vi "Motor_Plus_Impedance_controller.vi"() -> ()   [LabVIEW 2016]
uses:
  <vilib>/Platform/TimedLoop/XDataNode/timing_clust.ctl
  <vilib>/Platform/TimedLoop/XDataNode/nitl_modes.ctl
  <vilib>/Platform/TimedLoop/XDataNode/wakeup.ctl
  <vilib>/Platform/TimedLoop/XDataNode/loadnilvce.vi
  <vilib>/Motion/Express/_s/nimc.ax.power.power.axis.vi
  <vilib>/Motion/Express/_s/nimc.fb.stopMove.stop.axis.modeDecelerate.vi
  <vilib>/Motion/Express/_s/nimc.fb.read.readExecutionData.axis.vi
  <vilib>/Motion/Express/_s/nimc.fb.straightLineMove.startStraightLineMove.axis.modeAbsolute.0.vi
  <vilib>/Motion/Express/_s/nimc.ex.power.power.axis.vi
  <vilib>/platform/TimedLoop/XDataNode/XDataNode.xnode
  <vilib>/Motion/BlockNode/FB.NIMotion.xnode
  <vilib>/Platform/TimedLoop/XDataNode/XDNodeRunTimeDep.lvlib
panel:
  out "Torque":dbl(knob) scale=0.0..10.0
  out "Position":dbl(knob) scale=0.0..10.0
  out "Velocity":dbl(knob) scale=0.0..10.0
  out "Load Cell":dbl(knob) scale=0.0..10.0
  in  "desired motor\nposition":dbl
  in  "Move to Position?":bool
  out "Load cell, V":dbl format="%.3f"
  out "motor torque, Nm":dbl format="%.3f"
  out "motor velocity, rev/s":dbl format="%.3f"
  out "motor position, rev":dbl format="%.3f"
  in  "STOP VI":bool
  in  "Enable Axis \nControl":bool
  in  "Enable Motor \nDrive":bool
  in  "EMERGENCY MOTOR STOP":bool
  # "Raw Data from System"
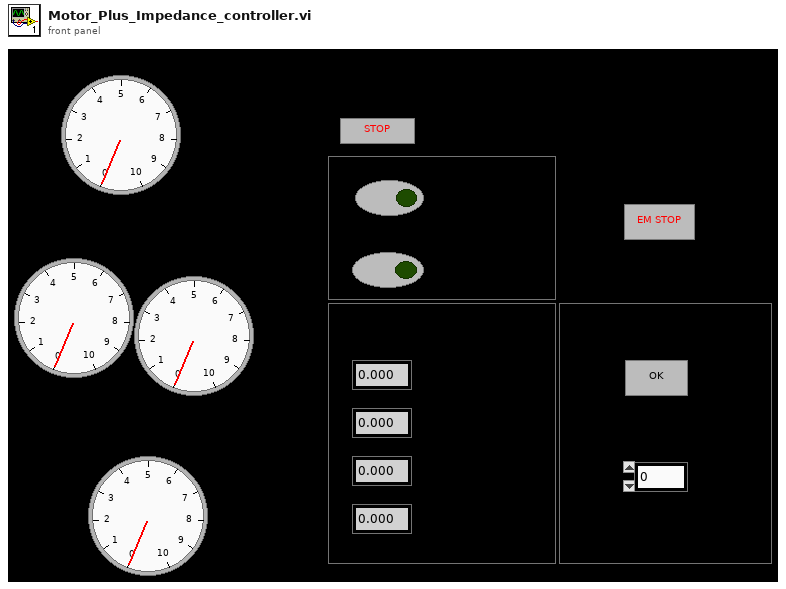
[diagram p1: front panel]
types:
  T1 = typedef "XDNodeRunTimeDep.lvlib/timing_clust.ctl" = cluster{"Expected End [f-1]":u64, "Actual End [f-1]":u64, "Finished Late? [f-1]":bool, "Expected End [i-1]":u64, "Actual End [i-1]":u64, "Finished Late? [i-1]":bool, "Expected Start [i]":u64, "Actual Start [i]":u64, "Expected Start [f]":u64, "Actual Start [f]":u64, "Source Name":string, "Structure Name":string, "Period":i64, "Deadline":i64, "Offset":i64, "Start":i64, "Priority":i32, "Timeout":i32, "Mode":T2, "Wakeup Reason":T3, "Error":errorcluster, "Source Type":string, "Secondary Source Type":string, "Global End Time":u64, "Global Start Time":u64, "Frame Duration":u64, "Iteration Duration":u64, "Assigned CPU":i32, "I/O Scan Engine Mode":u32}
  T2 = typedef "XDNodeRunTimeDep.lvlib/nitl_modes.ctl" = enum32{"No Change", "Process missed periods, maintain original phase", "Discard missed periods, maintain original phase", "Process missed periods, ignore original phase", "Discard missed periods, ignore original phase"}
  T3 = typedef "XDNodeRunTimeDep.lvlib/wakeup.ctl" = enum32{"Normal", "Aborted", "Asynchronous wakeup", "Timing source error", "Timed loop error", "Timeout"}
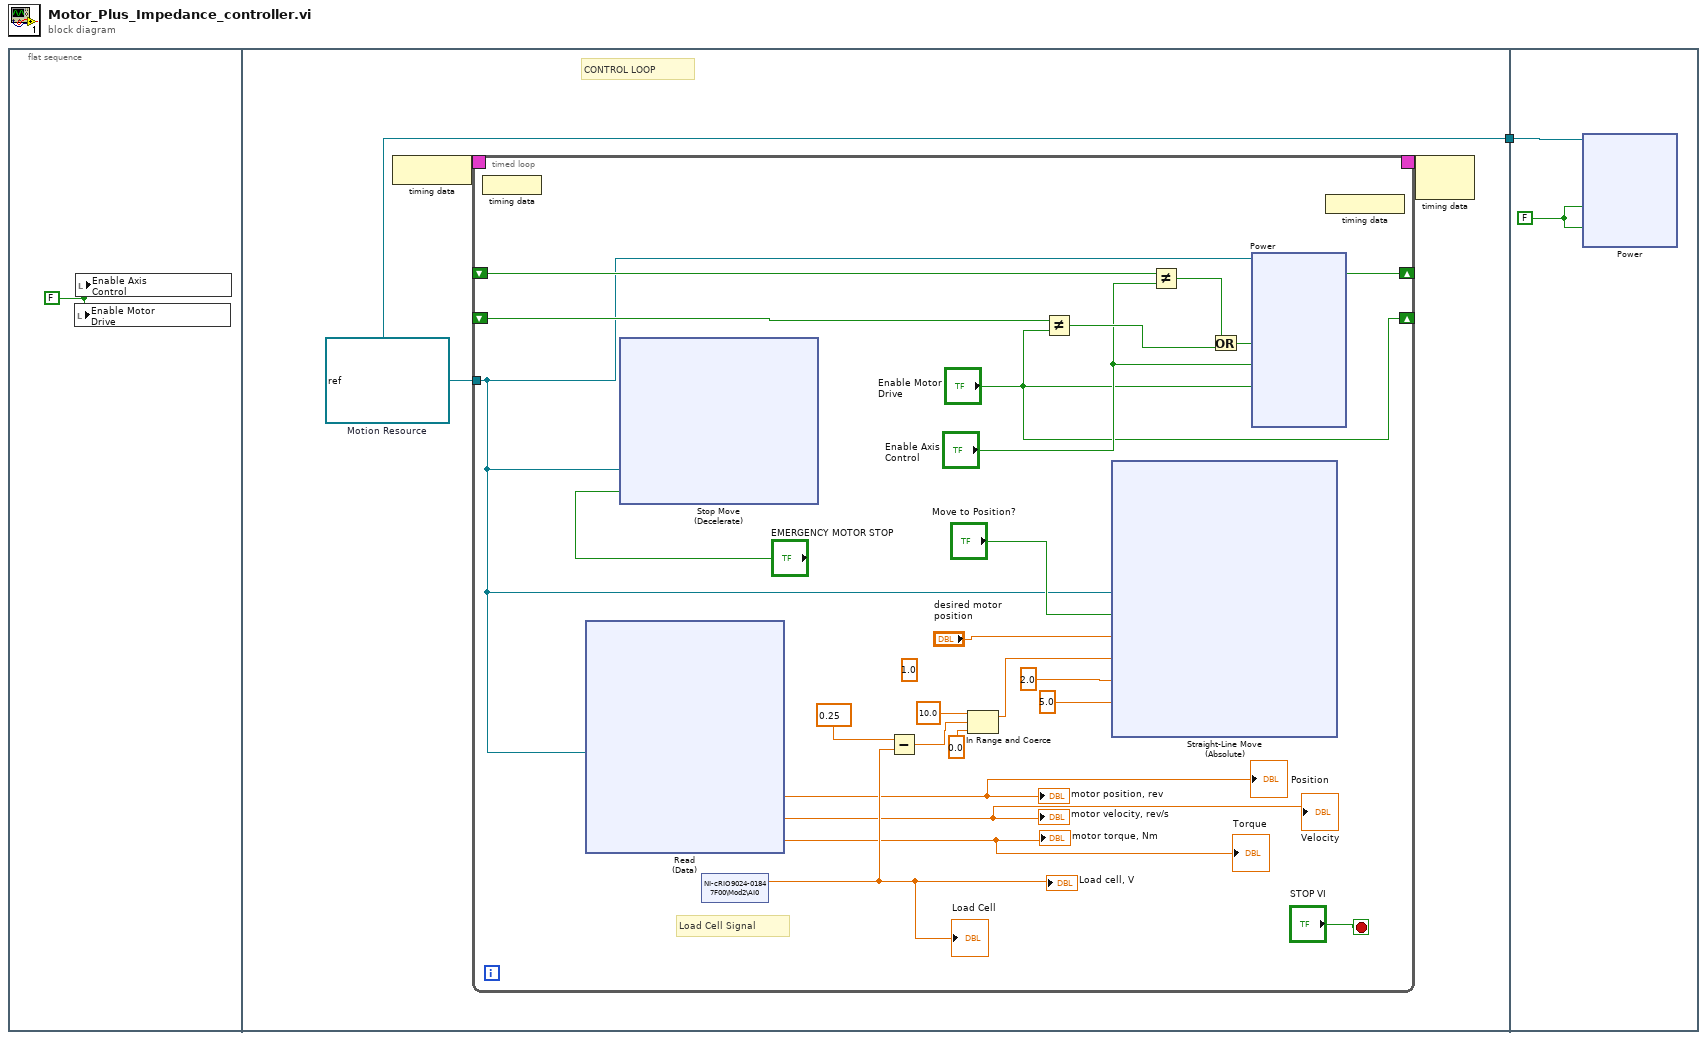
[diagram p0: block diagram]
diagram:
  n1 = flat-sequence {
    tunnel: [w5] -> w1
    tunnel: w1 -> [w96]
    frame #0 {
      w2 = FALSE
      n2 = local write "Enable Motor \nDrive"(w2) -> ()
      n3 = local write "Enable Axis \nControl"(w2) -> ()
    }
    frame #1 {
      w5 = refnum<k21> "nism://NI-cRIO9024-01847F00/Axis 1"  # Motion Resource
      # "CONTROL LOOP"
      n4 = node-c288() -> (w4:T1)
      n5 = timed-loop {
        tunnel: w5 -> [w16]
        timing: w4 -> [_]
        timing-out: [_] -> w3
        shift-right: ["Enable Axis \nControl"] -> _
        shift-left: _ -> [w24]
        shift-right: ["Enable Motor \nDrive"] -> _
        shift-left: _ -> [w23]
        stop <- "STOP VI" stop-if-true
        (unwired) 1.0
        # "Load Cell Signal"
        n6 = node-c288() -> ()  [unwired: 1 in]
        n7 = xnode "Read\n(Data)"("resource"=w16) -> ("position"=→"motor position, rev" →"Position":dbl, "torque"=→"motor torque, Nm" →"Torque":dbl, "velocity"=→"motor velocity, rev/s" →"Velocity":dbl)  [unwired: 1 in, 3 out]
        n8 = xnode "Stop Move\n(Decelerate)"("resource"=w16, "execute"="EMERGENCY MOTOR STOP") -> ()  [unwired: 1 in, 3 out]
        n9 = shared-variable "NI-cRIO9024-01847F00\\Mod2\\AI0"() -> (w9:dbl)  [unwired: 1 in, 1 out]
        "Load cell, V" <- w9
        "Load Cell" <- w9
        n10 = Subtract(x=0.25, y=w9) -> (x-y=w11:dbl)
        n11 = In Range and Coerce(upper limit=10.0, x=w11, lower limit=0.0) -> (coerced(x)=w10:dbl)  [unwired: 1 out]
        n12 = Not Equal?(x=w23, y="Enable Motor \nDrive") -> (x != y?=w21:bool)
        n13 = xnode "Straight-Line Move\n(Absolute)"("resource"=w16, "execute"="Move to Position?", "position"="desired motor\nposition", "velocity"=w10, "acceleration"=2.0, "deceleration"=5.0) -> ()  [unwired: 1 in, 3 out]
        n14 = Not Equal?(x=w24, y="Enable Axis \nControl") -> (x != y?=w22:bool)
        n15 = Or(x=w22, y=w21) -> (x .or. y?=w20:bool)
        n16 = xnode ("Power")("execute"=w20, "enable axis"="Enable Axis \nControl", "enable drive"="Enable Motor \nDrive", "resource"=w16) -> ()  [unwired: 1 in, 6 out]
        n17 = node-c288() -> ()  [unwired: 1 out]
      }
      n18 = node-c288(w3) -> ()  [unwired: 1 out]
    }
    frame #2 {
      w97 = FALSE
      n19 = xnode ("Power")("enable axis"=w97, "enable drive"=w97, "resource"=w96) -> ()  [unwired: 1 in, 2 out]
    }
  }
